vi "WavesAsyncCall.vi"(9 "数组":refnum<vi>[](array[refnum]), 10 "WaveformGraph输入":refnum<vi>, 11 "VISA资源名称输入":refnum<visa-resource-name>) -> (3 "VISA资源名称输出":refnum<visa-resource-name>)   [LabVIEW 2018]
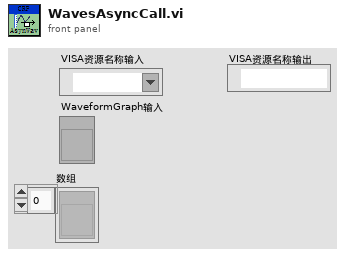
[diagram p1: front panel]
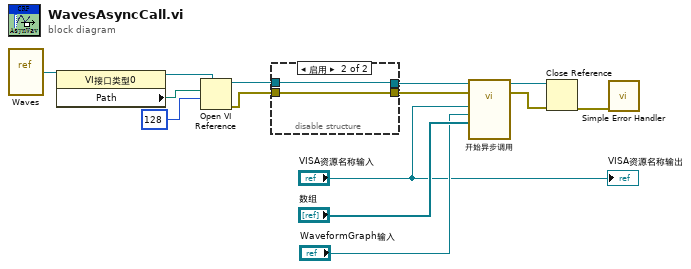
[diagram p0: block diagram]
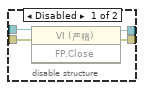
[diagram p2: hidden frame]
diagram:
  n1 = vi-ref "Waves.vi"() -> (w11:refnum<vi>)
  n2 = property class="VI接口类型0"(reference=w11) -> (reference out=w12:refnum<vi>, "Path"=w13:path)  [unwired: 1 in, 1 out]
  n3 = Open VI Reference(type specifier VI Refnum (for type only)=w12, vi path=w13, options=128 ("选项")) -> (vi reference=w10:refnum<vi>, error out=w5:errorcluster)  [unwired: 3 in]
  n4 = disable-structure shown="启用" {
    disable-tunnel: w10 -> [w18 w20]
    disable-tunnel: [w17 w19] -> w7
    disable-tunnel: [w16 w20] -> w6
    disable-tunnel: w5 -> [w15 w19]
    frame Disabled {
      n5 = invoke class="VI (严格)" method="FP.Close"(reference=w18, error in=w15) -> (reference out=w16:refnum<vi>, error out=w17:errorcluster)  [unwired: 1 in, 1 out]
    }
    frame Enabled {
    }
  }
  n6 = call-by-ref "开始异步调用"(reference=w6, error in=w7, "通道使能引用数组"="数组", "波形图"="WaveformGraph输入", "VISA资源名称输入"="VISA资源名称输入") -> (reference out=w4:refnum<vi>, error out=w3:errorcluster)  [unwired: 7 in, 2 out]
  n7 = Close Reference(reference=w4, error in (no error)=w3) -> (error out=w2:errorcluster)
  n8 = call <vilib>:"Simple Error Handler.vi"("error in (no error)"=w2) -> ()  [unwired: 4 in, 5 out]
  "VISA资源名称输出" <- "VISA资源名称输入"
